vi "delete tag select.vi"(8 "error in":errorcluster, 10 "tag selecct name":string, 11 "tag select module configuration in":refnum<class "tag select module configuration.lvclass">) -> (0 "error out":errorcluster, 2 "deleted channels":refnum<class "TBM channel.lvclass">[](array[class]), 3 "tag select module configuration out":refnum<class "tag select module configuration.lvclass">)   [LabVIEW 2013, in "tag select module configuration.lvclass"]
uses:
  tag select module configuration.lvclass
  <vilib>/NI/Tag Bus Module Framework/channel/TBM channel.lvclass
  tag select module configuration.lvclass/tag select module configuration.ctl
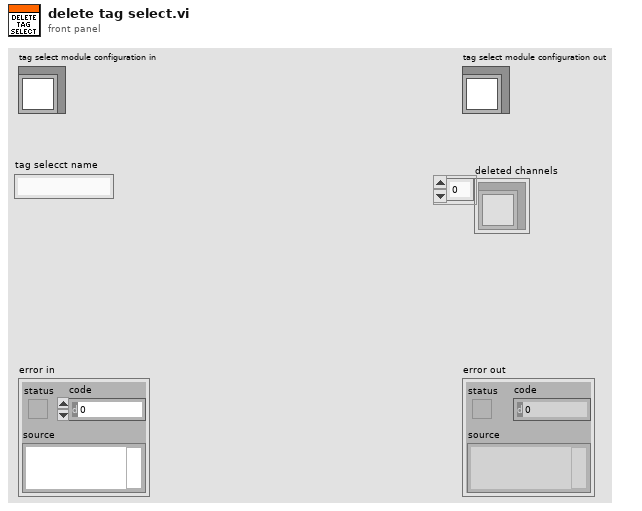
[diagram p1: front panel]
types:
  T1 = typedef "tag select module configuration.lvclass/tag select configuration.ctl" = cluster{"tag select name":string, "data type":T2, "channel":refnum<class "TBM channel.lvclass">}
  T2 = typedef "tag bus.lvlib/tag descriptor.lvclass/Data Type.ctl" = enum16{"Double", "Single", "I64", "I32", "I16", "I8", "U64", "U32", "U16", "U8", "Boolean", "String", "Array of Double", "Array of Single", "Array of I64", "Array of I32", "Array of I16", "Array of I8", "Array of U64", "Array of U32", "Array of U16", "Array of U8", "Array of Boolean", "Array of String"}
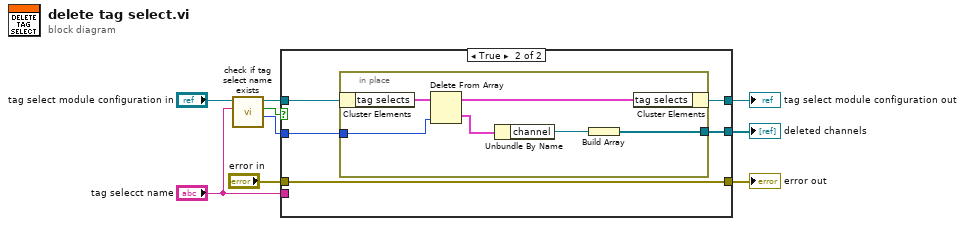
[diagram p0: block diagram]
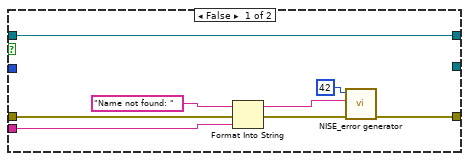
[diagram p2: hidden frame]
diagram:
  n1 = call "check if tag select name exists.vi"("name to locate"="tag selecct name", "tag select module configuration in"="tag select module configuration in") -> ("index"=w2:i32, "found?"=w6:bool, "tag select module configuration out"=w4:refnum<class "tag select module configuration.lvclass">)  [unwired: 6 in, 1 out]
  n2 = case shown="True" w6 {
    tunnel: [w16 w20] -> w8
    tunnel: "error in" -> [w17 w20]
    tunnel: [w11 w21] -> w5
    tunnel: w4 -> [w11 w22]
    tunnel: [_ w19] -> w3
    tunnel: w2 -> [_ w18]
    tunnel: "tag selecct name" -> [w10 _]
    frame False {
      n3 = Format Into String(initial string="Name not found: " ("append error message"), error in=w17, w10) -> (resulting string=w12:string, error out=w14:errorcluster)  [unwired: 1 in]
      n4 = call <vilib>:"NISE_error generator.vi"("error in"=w14, "append error message"=w12, "error code (0)"=42) -> ("error out"=w16:errorcluster)  [unwired: 6 in]
    }
    frame True {
      n5 = in-place {
        in-place-border: [w24] -> w19
        in-place-border: w18 -> [w26]
        n6 = in-place-cluster #1(w22) -> ("tag selects"=w28:T1[])
        n7 = Delete From Array(array=w28, index=w26) -> (deleted portion=w25:T1, array with subset deleted=w27:T1[])  [unwired: 1 in]
        n8 = Unbundle By Name(w25) -> ("channel"=w23:refnum<class "TBM channel.lvclass">)
        n9 = Build Array(w23) -> (w24:refnum<class "TBM channel.lvclass">[])
        n10 = in-place-cluster #1("tag selects"=w27) -> (w21:refnum<class "tag select module configuration.lvclass">)
      }
    }
  }
  "error out" <- w8
  "tag select module configuration out" <- w5
  "deleted channels" <- w3
